vi "ALTS-2015 Station Occupancy Status.vi"(8 "error in":errorcluster) -> (0 "error out":errorcluster, 2 "Available Station":T1, 3 "Station Unavailable":bool)   [LabVIEW 2013]
uses:
  Controls/ALTS-2015 Station Cluster.ctl
  Controls/ALTS-2015 LV2GBL Station Info Options.ctl
  Controls/ALTS-2015 LV2GBL Options.ctl
panel:
  # "ALTS-2015\nStation Occupancy Status"
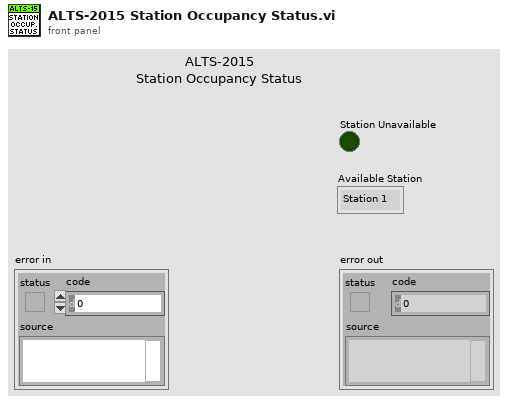
[diagram p1: front panel]
types:
  T1 = typedef "ALTS-2015 Station Cluster.ctl" = enum16{"Station 1", "Station 2", "Station 3", "Station 4"}
  T2 = typedef "ALTS-2015 LV2GBL Options.ctl" = enum16{"Read all", "Write all"}
  T3 = typedef "ALTS-2015 LV2GBL Station Info Options.ctl" = enum16{"Init", "Read", "Read All", "Write Sensor ID", "Write  Work Order", "Write Serial Number", "Write Test Data", "Write Station Status", "Write Station Occupancy", "Write Station Test Type", "Write Rerun", "Write Load Decision", "Write Robot Action", "Clear All", "Clear Test Result"}
  T4 = typedef "ALTS-2015 Station Details.ctl" = cluster{"Station Number":string, "Work Order Number":string, "Sensor Name":string, "Pressure (PSI)":string, "Flow (SCCM)":string, "Test Time ":string, "Test Result":string, "Serial Number":string, "Station Status":T5, "SW assigned UUT":bool, "Rerun Count":i32, "Test Type":i32, "Load Decision":i32, "Robot Action":T6}
  T5 = typedef "ALTS-2015 Status Ring Indicator.ctl" = u16
  T6 = typedef "ALTS-2015 Robot Actions.ctl" = enum16{"Loading...", "Unloading...", "Reruning...", "No Action"}
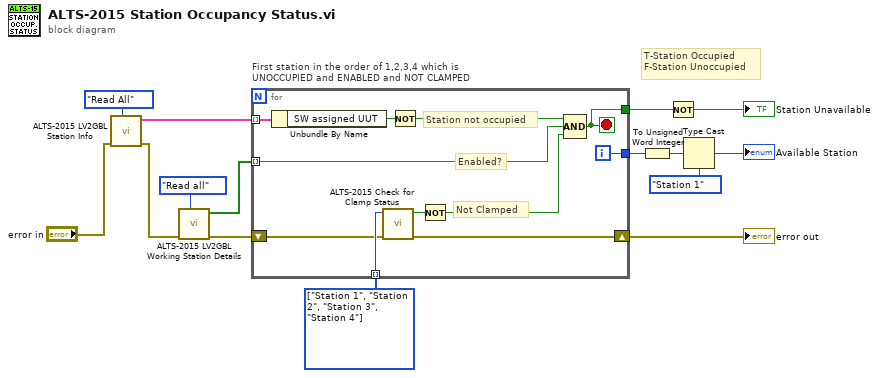
[diagram p0: block diagram]
diagram:
  w3 = T1[] [enum."Station 1", enum."Station 2", enum."Station 3", enum."Station 4"] items=["Station 1", "Station 2", "Station 3", "Station 4"]
  # "T-Station Occupied\nF-Station Unoccupied"
  n1 = call "ALTS-2015 LV2GBL Station Info.vi"("Options"=ALTS-2015_LV2GBL_Station_Info_Options."Read All", "error in"="error in") -> ("error out"=w11:errorcluster, "Station Info Array"=w14:T4[])  [unwired: 7 in, 1 out]
  n2 = call "ALTS-2015 LV2GBL Working Station Details.vi"("Options"=ALTS-2015_LV2GBL_Options."Read all", "error in"=w11) -> ("error out"=w2:errorcluster, "Station  Enable Array"=w10:bool[])  [unwired: 8 in]
  n3 = for "First station in the order of 1,2,3,4 which is\nUNOCCUPIED and ENABLED and NOT CLAMPED" {
    tunnel: w14 -> [w26] mode=indexing
    tunnel: w10 -> [w23] mode=indexing
    tunnel: [w22] -> w8
    tunnel: [w21] -> w9
    tunnel: w3 -> [w20] mode=indexing
    shift-right: [w18] -> w1
    shift-left: w2 -> [w19]
    i -> [w22]
    stop <- w21 stop-if-true
    # "Station not occupied"
    # "Enabled?"
    # "Not Clamped"
    n4 = Unbundle By Name(w26) -> ("SW assigned UUT"=w25:bool)
    n5 = call "ALTS-2015 Check for Clamp Status .vi"("error in (no error)"=w19, "Station Cluster"=w20) -> ("error out"=w18:errorcluster, "Clamp?"=w17:bool)  [unwired: 8 in]
    n6 = Not(x=w25) -> (.not. x?=w24:bool)
    n7 = Not(x=w17) -> (.not. x?=w16:bool)
    n8 = Compound Arithmetic op=AND(w24, w23, w16) -> (w21:bool)
  }
  "error out" <- w1
  n9 = To Unsigned Word Integer(number=w8) -> (unsigned 16bit integer=w6:u16)
  n10 = Not(x=w9) -> (.not. x?=→"Station Unavailable":bool)
  n11 = Type Cast(type=ALTS-2015_Station_Cluster."Station 1" ("Station Cluster"), x=w6) -> (*(type *) &x=→"Available Station":T1)
